vi "TempAlgoTest (SubVI).vi"(0 "Temp":refnum<vi>, 1 "Speed Ind":dbl format="%#_13g", 2 "Motor Speed RPM":refnum<vi>, 3 "Round":T1(ring), 4 "Temp Up In":dbl format="%#_13g", 5 "error in (no error)":errorcluster, 6 "String in":refnum<vi>, 7 "Temp Goal":dbl format="%#_13g", 8 "Stop":refnum<vi>, 9 "Speed Goal":dbl format="%#_13g", 10 "Stop BurnIn":refnum<vi>, 11 "AD Resistor Step":i32=9, 12 "Strin":string) -> (14 "Speed Pass/Fail":bool, 15 "Temp  Pass/Fail":dbl, 16 "Temp Up Out":dbl, 17 "Speed Pass/Fail":dbl, 18 "Temp Pass/Fail":bool, 19 "error out":errorcluster)   [LabVIEW 2017]
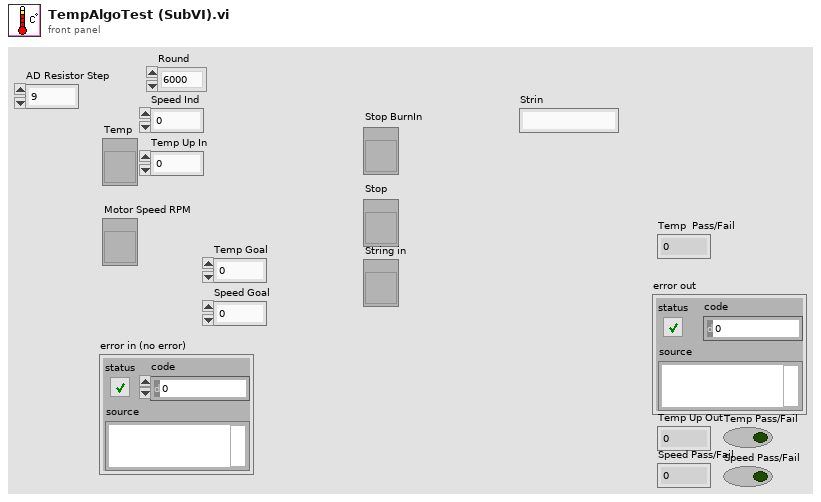
[diagram p1: front panel]
types:
  T1 = enum32{"6000", "11500", "15100", "11500-2", "6000-2"}
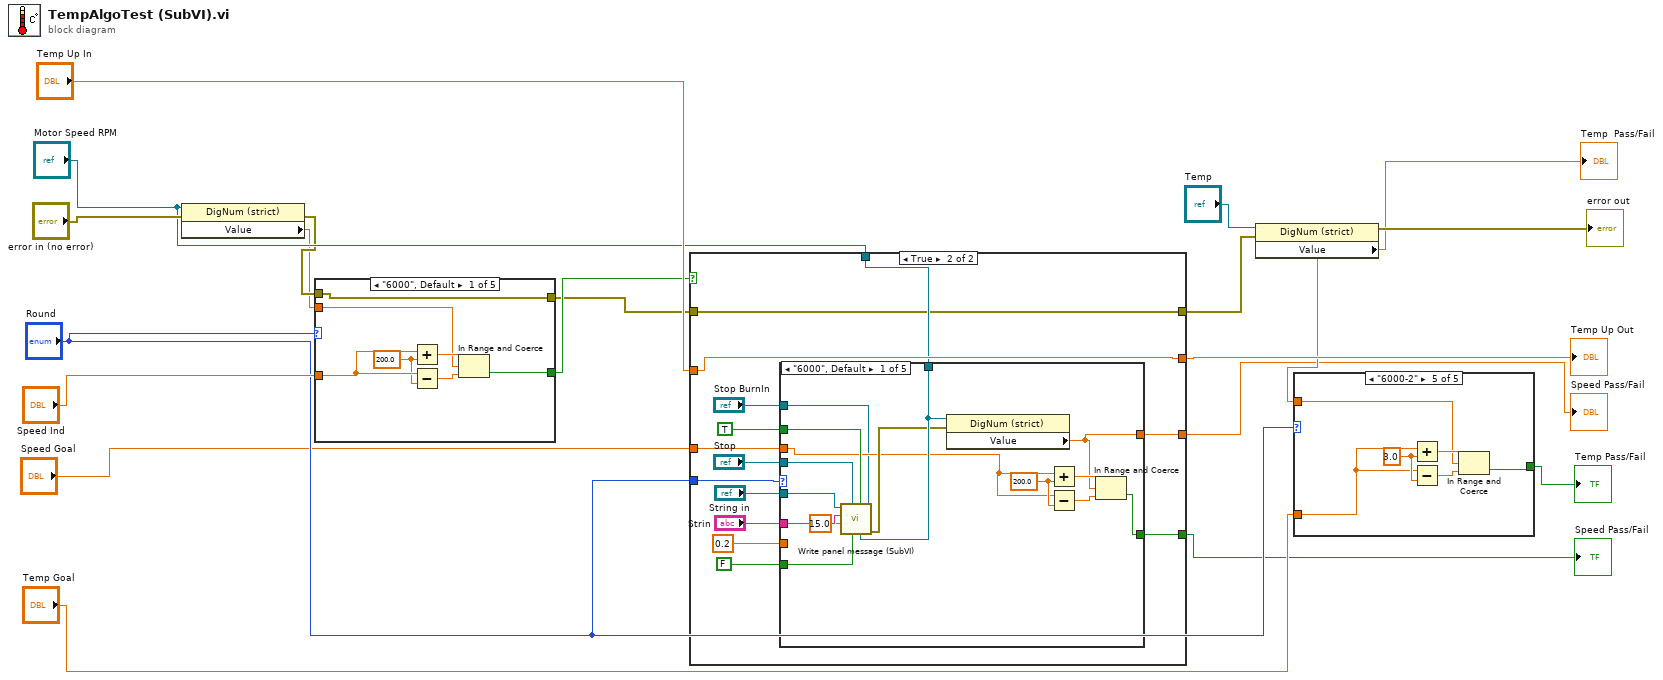
[diagram p0: block diagram]
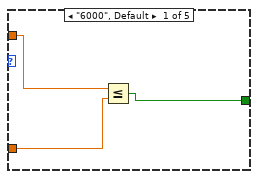
[diagram p2: hidden frame]
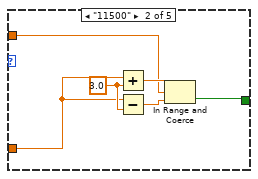
[diagram p3: hidden frame]
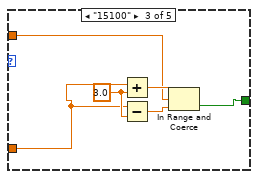
[diagram p4: hidden frame]
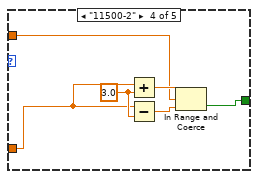
[diagram p5: hidden frame]
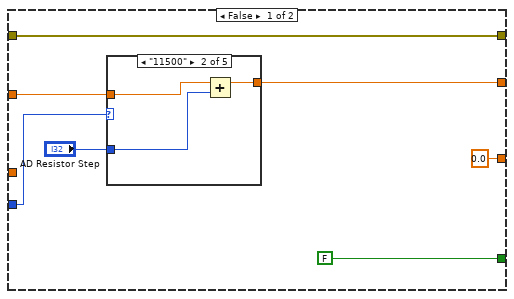
[diagram p6: hidden frame]
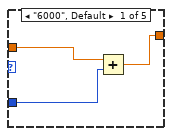
[diagram p7: hidden frame]
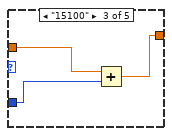
[diagram p8: hidden frame]
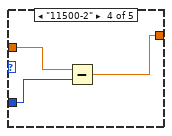
[diagram p9: hidden frame]
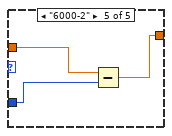
[diagram p10: hidden frame]
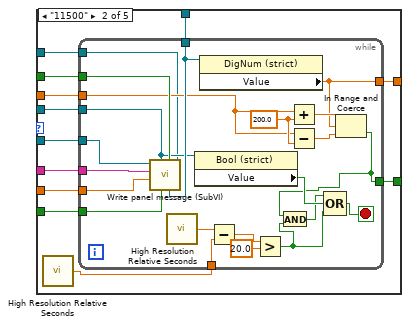
[diagram p11: hidden frame]
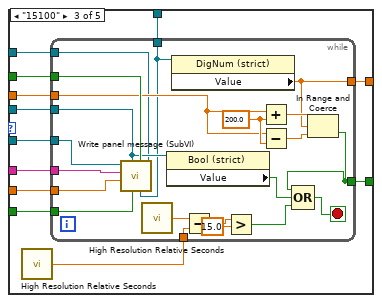
[diagram p12: hidden frame]
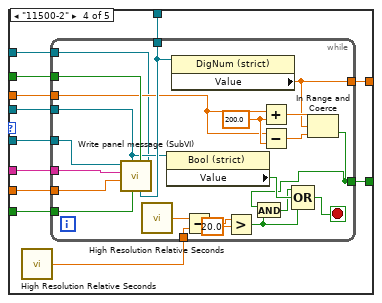
[diagram p13: hidden frame]
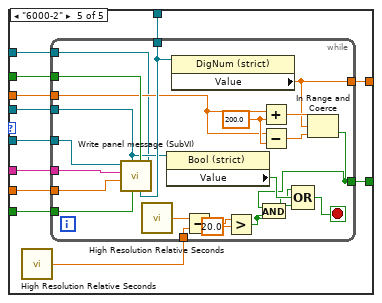
[diagram p14: hidden frame]
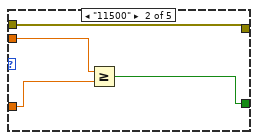
[diagram p15: hidden frame]
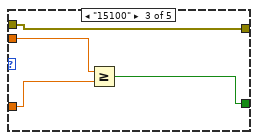
[diagram p16: hidden frame]
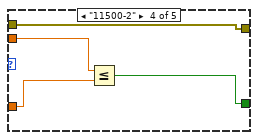
[diagram p17: hidden frame]
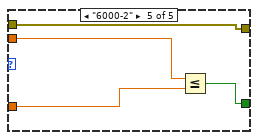
[diagram p18: hidden frame]
diagram:
  n1 = property class="DigNum (strict)"(reference="Motor Speed RPM", error in="error in (no error)") -> (error out=w6:errorcluster, "Value"=w3:dbl)  [unwired: 1 out]
  n2 = case shown="\"6000\", Default" "Round" {
    tunnel: w3 -> [w23 w30 w34 w38 w42]
    tunnel: "Speed Ind" -> [w24 w29 w33 w37 w41]
    tunnel: [w21 w28 w32 w36 w40] -> w14
    tunnel: w6 -> [w20 w27 w31 w35 w39]
    tunnel: [w20 w27 w31 w35 w39] -> w5
    frame "6000", Default {
      w22 = 200.0 ("y")
      n3 = Add(x=w24, y=w22) -> (x+y=w26:dbl)
      n4 = Subtract(x=w24, y=w22) -> (x-y=w25:dbl)
      n5 = In Range and Coerce(upper limit=w26, x=w23, lower limit=w25) -> (In Range?=w21:bool)  [unwired: 1 out]
    }
    frame "11500" {
      n6 = Greater Or Equal?(x=w30, y=w29) -> (x >= y?=w28:bool)
    }
    frame "15100" {
      n7 = Greater Or Equal?(x=w34, y=w33) -> (x >= y?=w32:bool)
    }
    frame "11500-2" {
      n8 = Less Or Equal?(x=w38, y=w37) -> (x <= y?=w36:bool)
    }
    frame "6000-2" {
      n9 = Less Or Equal?(x=w42, y=w41) -> (x <= y?=w40:bool)
    }
  }
  n10 = case shown="True" w14 {
    tunnel: "Temp Up In" -> [w49 w78]
    tunnel: [w48 w78] -> w13
    tunnel: "Motor Speed RPM" -> [_ w70]
    tunnel: "Round" -> [w44 w69]
    tunnel: [FALSE ("rpm 2") w68] -> w7
    tunnel: w5 -> [w46 w67]
    tunnel: [w46 w67] -> w4
    tunnel: "Speed Goal" -> [_ w66]
    tunnel: [0.0 ("Value") w65] -> w1
    frame False {
      n11 = case shown="\"11500\"" w44 {
        tunnel: w49 -> [w52 w55 w58 w61 w64]
        tunnel: [w51 w54 w57 w60 w63] -> w48
        tunnel: "AD Resistor Step" -> [w50 w53 w56 w59 w62]
        frame "6000", Default {
          n12 = Add(x=w52, y=w50) -> (x+y=w51:dbl)
        }
        frame "11500" {
          n13 = Add(x=w55, y=w53) -> (x+y=w54:dbl)
        }
        frame "15100" {
          n14 = Add(x=w58, y=w56) -> (x+y=w57:dbl)
        }
        frame "11500-2" {
          n15 = Subtract(x=w61, y=w59) -> (x-y=w60:dbl)
        }
        frame "6000-2" {
          n16 = Subtract(x=w64, y=w62) -> (x-y=w63:dbl)
        }
      }
    }
    frame True {
      n17 = case shown="\"6000\", Default" w69 {
        tunnel: "Stop BurnIn" -> [w79 w105 w139 w172 w206]
        tunnel: TRUE ("rpm 2") -> [w91 w104 w138 w171 w205]
        tunnel: FALSE ("PrintTime") -> [w89 w103 w137 w170 w204]
        tunnel: "Stop" -> [w92 w102 w136 w169 w203]
        tunnel: 0.2 ("Time to wait") -> [_ w101 w135 w168 w202]
        tunnel: "Strin" -> [w90 w100 w134 w167 w201]
        tunnel: "String in" -> [w93 w99 w133 w166 w200]
        tunnel: w70 -> [w88 w98 w132 w165 w199]
        tunnel: [w81 w95 w129 w162 w196] -> w68
        tunnel: w66 -> [w82 w97 w131 w164 w198]
        tunnel: [w80 w96 w130 w163 w197] -> w65
        frame "6000", Default {
          w85 = 200.0 ("y")
          n18 = call "Write panel message (SubVI).vi"("Stop BurnIn"=w79, 4:"rpm"=w88, 5:"rpm"=w91, "PrintTime"=w89, "Stop"=w92, "Time to wait"=15.0, "Strin"=w90, "String in"=w93) -> ("error out"=w87:errorcluster)  [unwired: 3 in]
          n19 = property class="DigNum (strict)"(reference=w88, error in=w87) -> ("Value"=w80:dbl)  [unwired: 2 out]
          n20 = Add(x=w82, y=w85) -> (x+y=w83:dbl)
          n21 = Subtract(x=w82, y=w85) -> (x-y=w84:dbl)
          n22 = In Range and Coerce(upper limit=w83, x=w80, lower limit=w84) -> (In Range?=w81:bool)  [unwired: 1 out]
        }
        frame "11500" {
          n23 = call <vilib>:"High Resolution Relative Seconds.vi"() -> ("relative seconds"=w94:dbl)
          n24 = while {
            tunnel: w105 -> [w106]
            tunnel: w104 -> [w127]
            tunnel: w103 -> [w126]
            tunnel: w102 -> [w121]
            tunnel: w101 -> [w125]
            tunnel: w100 -> [w124]
            tunnel: w99 -> [w123]
            tunnel: w98 -> [w122]
            tunnel: w97 -> [w117]
            tunnel: [w116] -> w96
            tunnel: [w107] -> w95
            tunnel: w94 -> [w112]
            stop <- w115 stop-if-true
            w120 = 200.0 ("y")
            n25 = call "Write panel message (SubVI).vi"("Stop BurnIn"=w106, 4:"rpm"=w122, 5:"rpm"=w127, "PrintTime"=w126, "Stop"=w121, "Time to wait"=w125, "Strin"=w124, "String in"=w123) -> ()  [unwired: 3 in, 1 out]
            n26 = call <vilib>:"High Resolution Relative Seconds.vi"() -> ("relative seconds"=w113:dbl)
            n27 = property class="Bool (strict)"(reference=w121) -> ("Value"=w114:bool)  [unwired: 1 in, 2 out]
            n28 = property class="DigNum (strict)"(reference=w122) -> ("Value"=w116:dbl)  [unwired: 1 in, 2 out]
            n29 = Subtract(x=w113, y=w112) -> (x-y=w111:dbl)
            n30 = Greater?(x=w111, y=20.0) -> (0:w109:bool)
            n31 = Add(x=w117, y=w120) -> (x+y=w118:dbl)
            n32 = Subtract(x=w117, y=w120) -> (x-y=w119:dbl)
            n33 = In Range and Coerce(upper limit=w118, x=w116, lower limit=w119) -> (In Range?=w107:bool)  [unwired: 1 out]
            n34 = And(x=w107, y=w109) -> (x .and. y?=w108:bool)
            n35 = Compound Arithmetic op=OR(w108, w114, w109) -> (w115:bool)
          }
        }
        frame "15100" {
          n36 = call <vilib>:"High Resolution Relative Seconds.vi"() -> ("relative seconds"=w128:dbl)
          n37 = while {
            tunnel: w139 -> [w140]
            tunnel: w138 -> [w160]
            tunnel: w137 -> [w159]
            tunnel: w136 -> [w155]
            tunnel: w135 -> [w158]
            tunnel: w134 -> [w157]
            tunnel: w133 -> [w156]
            tunnel: w132 -> [w141]
            tunnel: w131 -> [w151]
            tunnel: [w150] -> w130
            tunnel: [w148] -> w129
            tunnel: w128 -> [w145]
            stop <- w149 stop-if-true
            w154 = 200.0 ("y")
            n38 = call "Write panel message (SubVI).vi"("Stop BurnIn"=w140, 4:"rpm"=w141, 5:"rpm"=w160, "PrintTime"=w159, "Stop"=w155, "Time to wait"=w158, "Strin"=w157, "String in"=w156) -> ()  [unwired: 3 in, 1 out]
            n39 = call <vilib>:"High Resolution Relative Seconds.vi"() -> ("relative seconds"=w146:dbl)
            n40 = property class="Bool (strict)"(reference=w155) -> ("Value"=w147:bool)  [unwired: 1 in, 2 out]
            n41 = property class="DigNum (strict)"(reference=w141) -> ("Value"=w150:dbl)  [unwired: 1 in, 2 out]
            n42 = Subtract(x=w146, y=w145) -> (x-y=w144:dbl)
            n43 = Greater?(x=w144, y=15.0) -> (0:w142:bool)
            n44 = Add(x=w151, y=w154) -> (x+y=w152:dbl)
            n45 = Subtract(x=w151, y=w154) -> (x-y=w153:dbl)
            n46 = In Range and Coerce(upper limit=w152, x=w150, lower limit=w153) -> (In Range?=w148:bool)  [unwired: 1 out]
            n47 = Compound Arithmetic op=OR(w148, w147, w142) -> (w149:bool)
          }
        }
        frame "11500-2" {
          n48 = call <vilib>:"High Resolution Relative Seconds.vi"() -> ("relative seconds"=w161:dbl)
          n49 = while {
            tunnel: w172 -> [w173]
            tunnel: w171 -> [w194]
            tunnel: w170 -> [w193]
            tunnel: w169 -> [w188]
            tunnel: w168 -> [w192]
            tunnel: w167 -> [w191]
            tunnel: w166 -> [w190]
            tunnel: w165 -> [w189]
            tunnel: w164 -> [w184]
            tunnel: [w183] -> w163
            tunnel: [w174] -> w162
            tunnel: w161 -> [w179]
            stop <- w182 stop-if-true
            w187 = 200.0 ("y")
            n50 = call "Write panel message (SubVI).vi"("Stop BurnIn"=w173, 4:"rpm"=w189, 5:"rpm"=w194, "PrintTime"=w193, "Stop"=w188, "Time to wait"=w192, "Strin"=w191, "String in"=w190) -> ()  [unwired: 3 in, 1 out]
            n51 = call <vilib>:"High Resolution Relative Seconds.vi"() -> ("relative seconds"=w180:dbl)
            n52 = property class="Bool (strict)"(reference=w188) -> ("Value"=w181:bool)  [unwired: 1 in, 2 out]
            n53 = property class="DigNum (strict)"(reference=w189) -> ("Value"=w183:dbl)  [unwired: 1 in, 2 out]
            n54 = Subtract(x=w180, y=w179) -> (x-y=w178:dbl)
            n55 = Greater?(x=w178, y=20.0) -> (0:w175:bool)
            n56 = Add(x=w184, y=w187) -> (x+y=w185:dbl)
            n57 = Subtract(x=w184, y=w187) -> (x-y=w186:dbl)
            n58 = In Range and Coerce(upper limit=w185, x=w183, lower limit=w186) -> (In Range?=w174:bool)  [unwired: 1 out]
            n59 = And(x=w174, y=w175) -> (x .and. y?=w176:bool)
            n60 = Compound Arithmetic op=OR(w176, w181, w175) -> (w182:bool)
          }
        }
        frame "6000-2" {
          n61 = call <vilib>:"High Resolution Relative Seconds.vi"() -> ("relative seconds"=w195:dbl)
          n62 = while {
            tunnel: w206 -> [w207]
            tunnel: w205 -> [w228]
            tunnel: w204 -> [w227]
            tunnel: w203 -> [w222]
            tunnel: w202 -> [w226]
            tunnel: w201 -> [w225]
            tunnel: w200 -> [w224]
            tunnel: w199 -> [w223]
            tunnel: w198 -> [w218]
            tunnel: [w217] -> w197
            tunnel: [w210] -> w196
            tunnel: w195 -> [w213]
            stop <- w216 stop-if-true
            w221 = 200.0 ("y")
            n63 = call "Write panel message (SubVI).vi"("Stop BurnIn"=w207, 4:"rpm"=w223, 5:"rpm"=w228, "PrintTime"=w227, "Stop"=w222, "Time to wait"=w226, "Strin"=w225, "String in"=w224) -> ()  [unwired: 3 in, 1 out]
            n64 = call <vilib>:"High Resolution Relative Seconds.vi"() -> ("relative seconds"=w214:dbl)
            n65 = property class="Bool (strict)"(reference=w222) -> ("Value"=w215:bool)  [unwired: 1 in, 2 out]
            n66 = property class="DigNum (strict)"(reference=w223) -> ("Value"=w217:dbl)  [unwired: 1 in, 2 out]
            n67 = Subtract(x=w214, y=w213) -> (x-y=w212:dbl)
            n68 = Greater?(x=w212, y=20.0) -> (0:w208:bool)
            n69 = Add(x=w218, y=w221) -> (x+y=w219:dbl)
            n70 = Subtract(x=w218, y=w221) -> (x-y=w220:dbl)
            n71 = In Range and Coerce(upper limit=w219, x=w217, lower limit=w220) -> (In Range?=w210:bool)  [unwired: 1 out]
            n72 = And(x=w210, y=w208) -> (x .and. y?=w209:bool)
            n73 = Compound Arithmetic op=OR(w209, w215, w208) -> (w216:bool)
          }
        }
      }
    }
  }
  "Temp Up Out" <- w13
  "Speed Pass/Fail" <- w7
  "Speed Pass/Fail" <- w1
  n74 = property class="DigNum (strict)"(reference="Temp", error in=w4) -> (error out=→"error out":errorcluster, "Value"=w12:dbl)  [unwired: 1 out]
  "Temp  Pass/Fail" <- w12
  n75 = case shown="\"6000-2\"" "Round" {
    tunnel: w12 -> [w230 w234 w240 w246 w252]
    tunnel: [w231 w232 w238 w244 w250] -> w10
    tunnel: "Temp Goal" -> [w229 w233 w239 w245 w251]
    frame "6000", Default {
      n76 = Less Or Equal?(x=w230, y=w229) -> (x <= y?=w231:bool)
    }
    frame "11500" {
      w235 = 3.0 ("y")
      n77 = Add(x=w233, y=w235) -> (x+y=w237:dbl)
      n78 = Subtract(x=w233, y=w235) -> (x-y=w236:dbl)
      n79 = In Range and Coerce(upper limit=w237, x=w234, lower limit=w236) -> (In Range?=w232:bool)  [unwired: 1 out]
    }
    frame "15100" {
      w241 = 3.0 ("y")
      n80 = Add(x=w239, y=w241) -> (x+y=w243:dbl)
      n81 = Subtract(x=w239, y=w241) -> (x-y=w242:dbl)
      n82 = In Range and Coerce(upper limit=w243, x=w240, lower limit=w242) -> (In Range?=w238:bool)  [unwired: 1 out]
    }
    frame "11500-2" {
      w247 = 3.0 ("y")
      n83 = Add(x=w245, y=w247) -> (x+y=w249:dbl)
      n84 = Subtract(x=w245, y=w247) -> (x-y=w248:dbl)
      n85 = In Range and Coerce(upper limit=w249, x=w246, lower limit=w248) -> (In Range?=w244:bool)  [unwired: 1 out]
    }
    frame "6000-2" {
      w253 = 3.0 ("y")
      n86 = Add(x=w251, y=w253) -> (x+y=w255:dbl)
      n87 = Subtract(x=w251, y=w253) -> (x-y=w254:dbl)
      n88 = In Range and Coerce(upper limit=w255, x=w252, lower limit=w254) -> (In Range?=w250:bool)  [unwired: 1 out]
    }
  }
  "Temp Pass/Fail" <- w10
